vi "Get Instrument Alias.vi"(8 "error in (no error)":errorcluster, 11 "HMC8043 in":refnum<class "HMC8043.lvclass">) -> (0 "error out":errorcluster, 2 "Instrument Alias":string, 3 "HMC8043 out":refnum<class "HMC8043.lvclass">)   [LabVIEW 2023, in "HAF.lvlib" / "HMC8043.lvclass"]
doc: "Returns the alias name of the Instrument for this Driver that can be used to initiate a session. Must be implemented by Subclasses because there is no Visa Session available to obtain it from when it is needed.\n\nIt's not ideal: need to think of a better way of dealing with attached resources than hard-coded aliases which must match what was entered in NI-MAX."
uses:
  HMC8043.lvclass
  HMC8043.lvclass/HMC8043.ctl
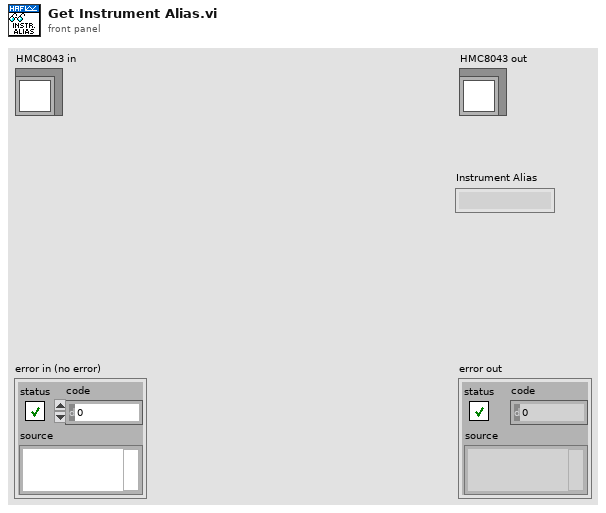
[diagram p1: front panel]
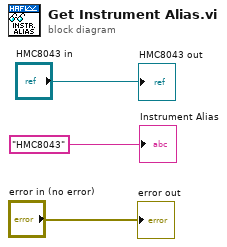
[diagram p0: block diagram]
diagram:
  "error out" <- "error in (no error)"
  "HMC8043 out" <- "HMC8043 in"
  "Instrument Alias" <- "HMC8043" ("Instrument Alias")
